vi "Zeit_seit_letztem_Aufruf.vi"(3 "mittlere Schleifenperiode":u32, 5 "Verstrichene Zeit [us]":u16) -> (0 "Zeit seit letztem Aufruf [us]":u32)   [LabVIEW 2013]
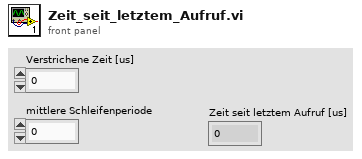
[diagram p1: front panel]
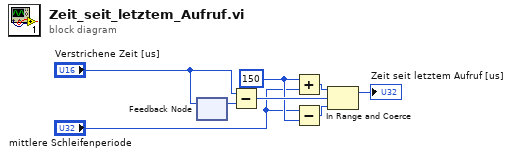
[diagram p0: block diagram]
diagram:
  w5 = u16 150 ("Iterationsdauer")
  n1 = feedback #1() -> (w3:u16)  [unwired: 1 in]
  n2 = feedback-in #1("Verstrichene Zeit [us]") -> ()
  n3 = Subtract(x="Verstrichene Zeit [us]", y=w3) -> (x-y=w8:u16)
  n4 = Add(x=w5, y="mittlere Schleifenperiode") -> (x+y=w7:u32)
  n5 = Subtract(x="mittlere Schleifenperiode", y=w5) -> (x-y=w6:u32)
  n6 = In Range and Coerce(upper limit=w7, x=w8, lower limit=w6) -> (coerced(x)=→"Zeit seit letztem Aufruf [us]":u32)  [unwired: 1 out]
